vi "Write Settings To VI Controls.vi"(0 "Control In":refnum<vi>, 5 "Control Values":T1[](array[typedef]), 11 "error in":errorcluster) -> (4 "Control Out":refnum<vi>, 15 "error out":errorcluster)   [LabVIEW 2020]
uses:
  <vilib>/addons/analyzer/_analyzerctrls.llb/VIAnCtl Config Control Value.ctl
  <vilib>/Utility/Data Type/NI_Data Type.lvlib
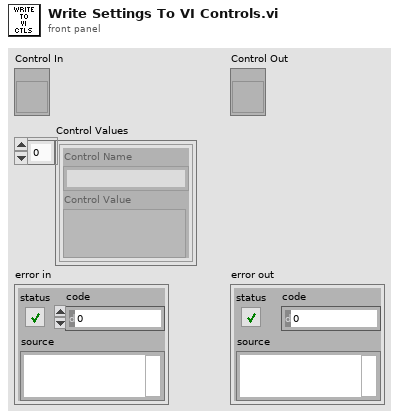
[diagram p1: front panel]
types:
  T1 = typedef "VIAnCtl Config Control Value.ctl" = cluster{"Control Name":string, "Control Value":variant}
  T2 = typedef "NI_Data Type.lvlib/Data Type.ctl" = enum8{"Invalid Type", "Void", "I8", "I16", "I32", "I64", "U8", "U16", "U32", "U64", "Single Float", "Double Float", "Extended Float", "Single Complex", "Double Complex", "Extended Complex", "Enum U8", "Enum U16", "Enum U32", "Enum U64", "Single Float With Unit", "Double Float With Unit", "Extended Float With Unit", "Single Complex with Unit", "Double Complex with Unit", "Extended Complex with Unit", "Boolean", "String", "Path", "Picture", "Tag", "Array", "Cluster", "Variant", "LV Variant", "Waveform", "Timestamp", "Digital Waveform", "Digital Data", "ExpressData", "Refnum", "External Data", "VI", "Poly VI", "LabVIEW Class Instance", "Fixed Point", "Set Collection", "Map Collection"}
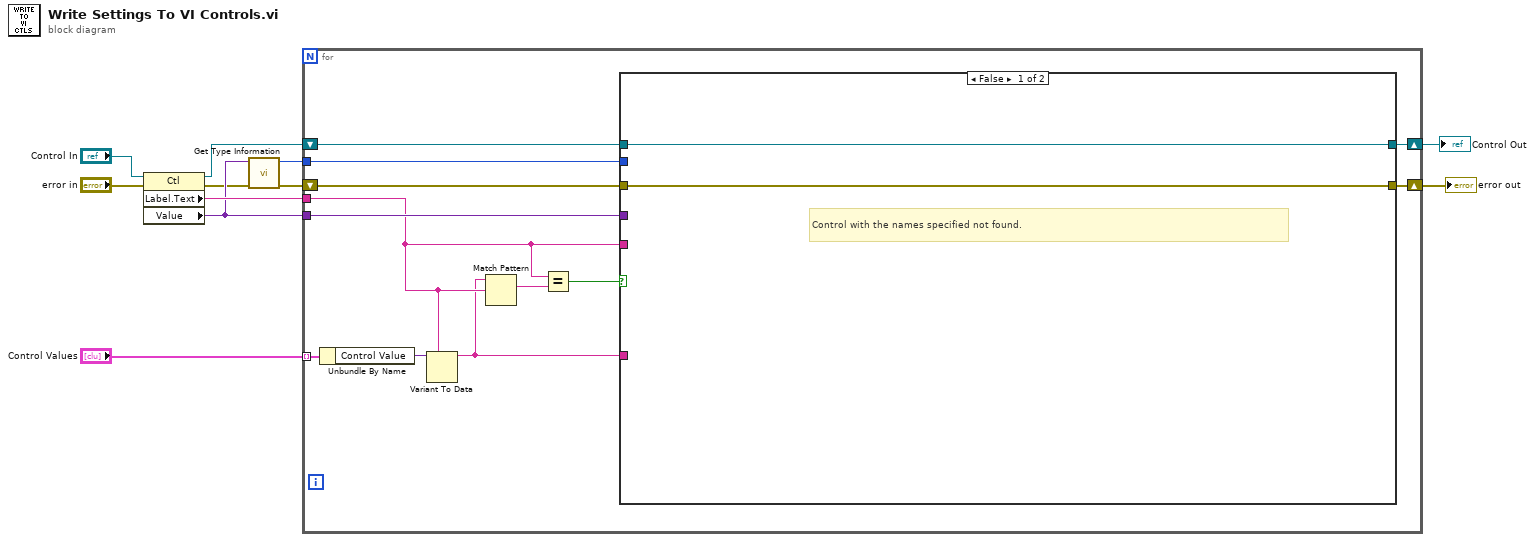
[diagram p0: block diagram]
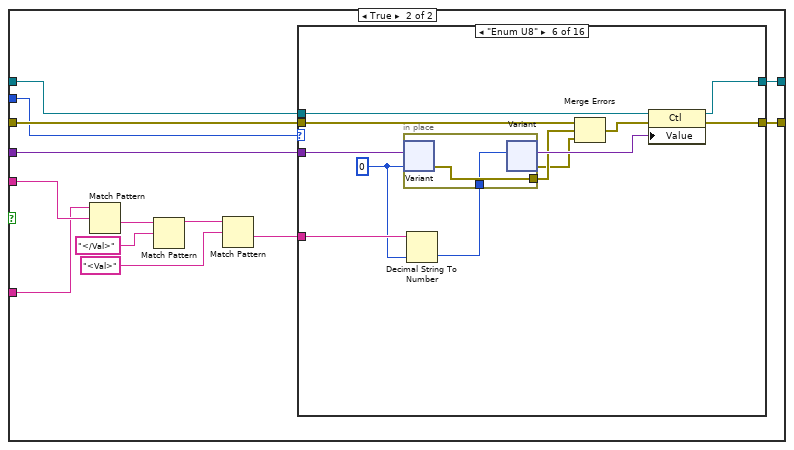
[diagram p2: hidden frame]
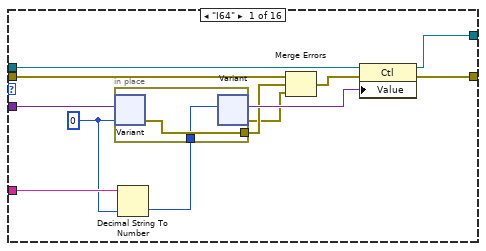
[diagram p3: hidden frame]
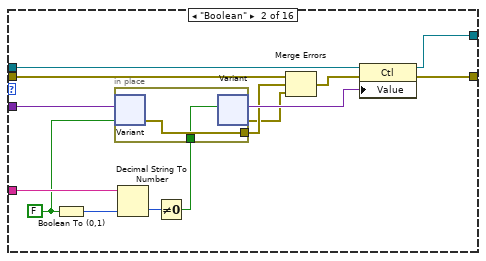
[diagram p4: hidden frame]
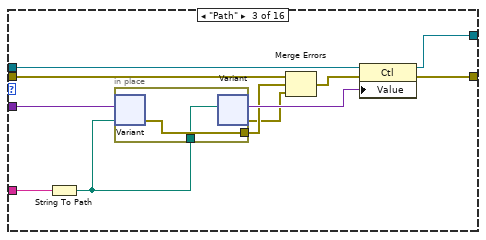
[diagram p5: hidden frame]
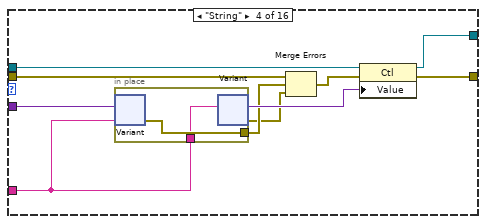
[diagram p6: hidden frame]
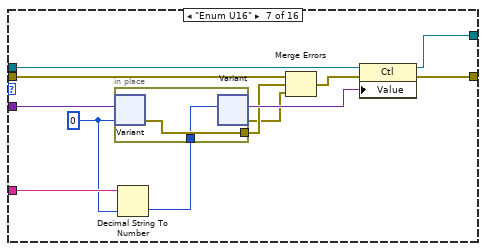
[diagram p8: hidden frame]
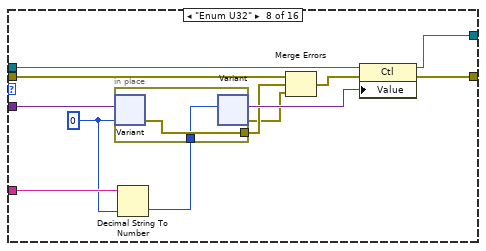
[diagram p9: hidden frame]
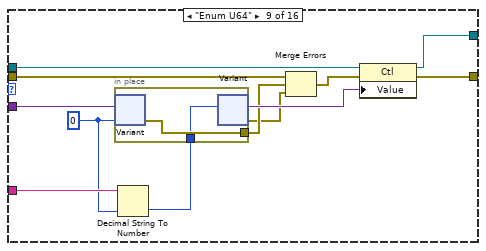
[diagram p10: hidden frame]
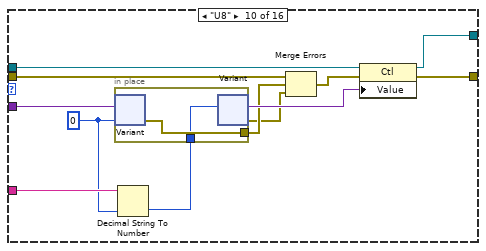
[diagram p11: hidden frame]
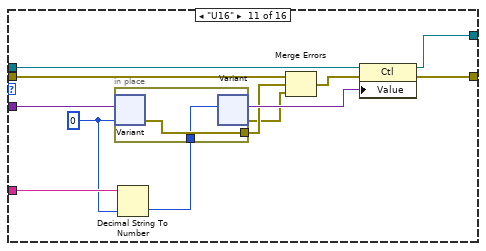
[diagram p12: hidden frame]
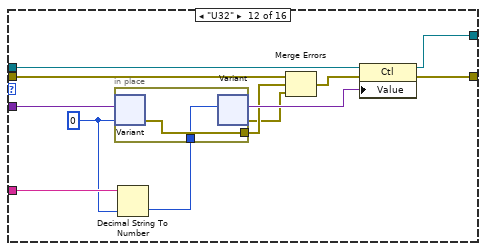
[diagram p13: hidden frame]
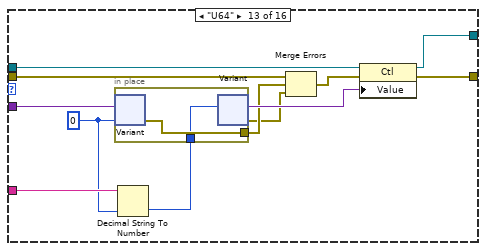
[diagram p14: hidden frame]
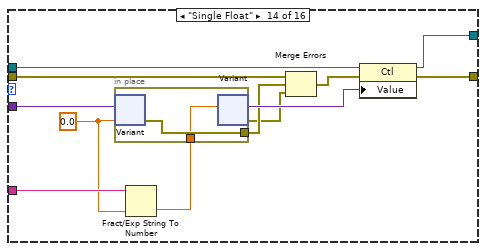
[diagram p15: hidden frame]
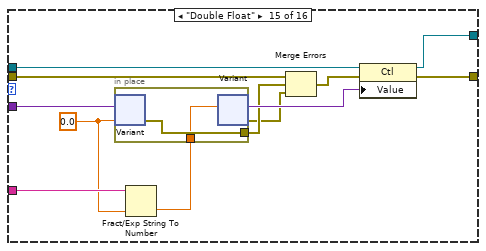
[diagram p16: hidden frame]
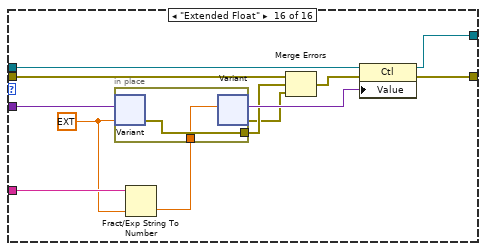
[diagram p17: hidden frame]
diagram:
  n1 = property class="Ctl"(reference="Control In", error in="error in") -> (reference out=w9:refnum<vi>, error out=w5:errorcluster, "Label.Text"=w10:string, "Value"=w6:variant)
  n2 = call <vilib>:"Get Type Information.vi"("error in (no error)"=w5, "variant"=w6) -> ("error out"=w7:errorcluster, "type"=w8:T2)  [unwired: 5 in, 3 out]
  n3 = for {
    shift-right: [w23] -> w2
    shift-left: w7 -> [w19]
    tunnel: "Control Values" -> [w17] mode=indexing
    tunnel: w6 -> [w22]
    tunnel: w8 -> [w21]
    tunnel: w10 -> [w13]
    shift-right: [w15] -> w1
    shift-left: w9 -> [w20]
    n4 = Unbundle By Name(w17) -> ("Control Value"=w14:variant)
    n5 = Variant To Data(type=w13, Variant=w14) -> (data=w12:string)  [unwired: 1 in, 1 out]
    n6 = Match Pattern(string=w12, regular expression=w13) -> (match substring=w16:string)  [unwired: 1 in, 3 out]
    n7 = Equal?(x=w13, y=w16) -> (x = y?=w18:bool)
    n8 = case shown="False" w18 {
      tunnel: [w25 w38] -> w23
      tunnel: w22 -> [_ w37]
      tunnel: w21 -> [_ w27]
      tunnel: w20 -> [w24 w36]
      tunnel: w19 -> [w25 w35]
      tunnel: w12 -> [_ w31]
      tunnel: w13 -> [_ w32]
      tunnel: [w24 w26] -> w15
      frame False {
        # "Control with the names specified not found."
      }
      frame True {
        n9 = Match Pattern(string=w31, regular expression=w32) -> (after substring=w34:string)  [unwired: 1 in, 3 out]
        n10 = Match Pattern(string=w34, regular expression="</Val>") -> (before substring=w30:string)  [unwired: 1 in, 3 out]
        n11 = Match Pattern(string=w30, regular expression="<Val>") -> (after substring=w28:string)  [unwired: 1 in, 3 out]
        n12 = case shown="\"Enum U8\"" w27 {
          tunnel: [w50 w66 w79 w91 w95 w107 w121 w135 w149 w163 w177 w191 w205 w219 w233 w247] -> w38
          tunnel: w37 -> [w49 w65 w78 w90 _ w106 w120 w134 w148 w162 w176 w190 w204 w218 w232 w246]
          tunnel: w36 -> [w48 w64 w77 w89 w94 w105 w119 w133 w147 w161 w175 w189 w203 w217 w231 w245]
          tunnel: w35 -> [w47 w63 w76 w88 w95 w104 w118 w132 w146 w160 w174 w188 w202 w216 w230 w244]
          tunnel: w28 -> [w46 w62 w71 w83 _ w103 w117 w131 w145 w159 w173 w187 w201 w211 w225 w239]
          tunnel: [w39 w53 w69 w82 w94 w96 w110 w124 w138 w152 w166 w180 w194 w208 w222 w236] -> w26
          frame "I64" {
            w40 = i64 0
            n13 = Decimal String To Number(string=w46, default (0L)=w40) -> (number=w41:i64)  [unwired: 1 in, 1 out]
            n14 = in-place {
              in-place-border: [w52] -> w43
              in-place-border: w41 -> [w51]
              n15 = in-place-variant #1(w49, w40) -> (w52:errorcluster)  [unwired: 1 out]
              n16 = in-place-variant #1(w51) -> (w45:variant, w42:errorcluster)
            }
            n17 = Merge Errors(w47, w43, w42) -> (w44:errorcluster)
            n18 = property class="Ctl"(reference=w48, error in=w44, "Value"=w45) -> (reference out=w39:refnum<vi>, error out=w50:errorcluster)
          }
          frame "Boolean" {
            w56 = FALSE ("Boolean")
            n19 = Boolean To (0,1)(Boolean=w56) -> (0, 1=w57:i16)
            n20 = Decimal String To Number(string=w62, default (0L)=w57) -> (number=w55:i16)  [unwired: 1 in, 1 out]
            n21 = Not Equal To 0?(x=w55) -> (x != 0?=w54:bool)
            n22 = in-place {
              in-place-border: [w68] -> w59
              in-place-border: w54 -> [w67]
              n23 = in-place-variant #2(w65, w56) -> (w68:errorcluster)  [unwired: 1 out]
              n24 = in-place-variant #2(w67) -> (w61:variant, w58:errorcluster)
            }
            n25 = Merge Errors(w63, w59, w58) -> (w60:errorcluster)
            n26 = property class="Ctl"(reference=w64, error in=w60, "Value"=w61) -> (reference out=w53:refnum<vi>, error out=w66:errorcluster)
          }
          frame "Path" {
            n27 = String To Path(string=w71) -> (path=w70:path)
            n28 = in-place {
              in-place-border: [w81] -> w73
              in-place-border: w70 -> [w80]
              n29 = in-place-variant #3(w78, w70) -> (w81:errorcluster)  [unwired: 1 out]
              n30 = in-place-variant #3(w80) -> (w75:variant, w72:errorcluster)
            }
            n31 = Merge Errors(w76, w73, w72) -> (w74:errorcluster)
            n32 = property class="Ctl"(reference=w77, error in=w74, "Value"=w75) -> (reference out=w69:refnum<vi>, error out=w79:errorcluster)
          }
          frame "String" {
            n33 = in-place {
              in-place-border: [w93] -> w85
              in-place-border: w83 -> [w92]
              n34 = in-place-variant #4(w90, w83) -> (w93:errorcluster)  [unwired: 1 out]
              n35 = in-place-variant #4(w92) -> (w87:variant, w84:errorcluster)
            }
            n36 = Merge Errors(w88, w85, w84) -> (w86:errorcluster)
            n37 = property class="Ctl"(reference=w89, error in=w86, "Value"=w87) -> (reference out=w82:refnum<vi>, error out=w91:errorcluster)
          }
          frame Default {
            # "Type not handled."
          }
          frame "Enum U8" {
            w97 = u8 0
            n38 = Decimal String To Number(string=w103, default (0L)=w97) -> (number=w98:u8)  [unwired: 1 in, 1 out]
            n39 = in-place {
              in-place-border: [w109] -> w100
              in-place-border: w98 -> [w108]
              n40 = in-place-variant #5(w106, w97) -> (w109:errorcluster)  [unwired: 1 out]
              n41 = in-place-variant #5(w108) -> (w102:variant, w99:errorcluster)
            }
            n42 = Merge Errors(w104, w100, w99) -> (w101:errorcluster)
            n43 = property class="Ctl"(reference=w105, error in=w101, "Value"=w102) -> (reference out=w96:refnum<vi>, error out=w107:errorcluster)
          }
          frame "Enum U16" {
            w111 = u16 0
            n44 = Decimal String To Number(string=w117, default (0L)=w111) -> (number=w112:u16)  [unwired: 1 in, 1 out]
            n45 = in-place {
              in-place-border: [w123] -> w114
              in-place-border: w112 -> [w122]
              n46 = in-place-variant #6(w120, w111) -> (w123:errorcluster)  [unwired: 1 out]
              n47 = in-place-variant #6(w122) -> (w116:variant, w113:errorcluster)
            }
            n48 = Merge Errors(w118, w114, w113) -> (w115:errorcluster)
            n49 = property class="Ctl"(reference=w119, error in=w115, "Value"=w116) -> (reference out=w110:refnum<vi>, error out=w121:errorcluster)
          }
          frame "Enum U32" {
            w125 = u32 0
            n50 = Decimal String To Number(string=w131, default (0L)=w125) -> (number=w126:u32)  [unwired: 1 in, 1 out]
            n51 = in-place {
              in-place-border: [w137] -> w128
              in-place-border: w126 -> [w136]
              n52 = in-place-variant #7(w134, w125) -> (w137:errorcluster)  [unwired: 1 out]
              n53 = in-place-variant #7(w136) -> (w130:variant, w127:errorcluster)
            }
            n54 = Merge Errors(w132, w128, w127) -> (w129:errorcluster)
            n55 = property class="Ctl"(reference=w133, error in=w129, "Value"=w130) -> (reference out=w124:refnum<vi>, error out=w135:errorcluster)
          }
          frame "Enum U64" {
            w139 = u64 0
            n56 = Decimal String To Number(string=w145, default (0L)=w139) -> (number=w140:u64)  [unwired: 1 in, 1 out]
            n57 = in-place {
              in-place-border: [w151] -> w142
              in-place-border: w140 -> [w150]
              n58 = in-place-variant #8(w148, w139) -> (w151:errorcluster)  [unwired: 1 out]
              n59 = in-place-variant #8(w150) -> (w144:variant, w141:errorcluster)
            }
            n60 = Merge Errors(w146, w142, w141) -> (w143:errorcluster)
            n61 = property class="Ctl"(reference=w147, error in=w143, "Value"=w144) -> (reference out=w138:refnum<vi>, error out=w149:errorcluster)
          }
          frame "U8" {
            w153 = u8 0 ("Numeric")
            n62 = Decimal String To Number(string=w159, default (0L)=w153) -> (number=w154:u8)  [unwired: 1 in, 1 out]
            n63 = in-place {
              in-place-border: [w165] -> w156
              in-place-border: w154 -> [w164]
              n64 = in-place-variant #9(w162, w153) -> (w165:errorcluster)  [unwired: 1 out]
              n65 = in-place-variant #9(w164) -> (w158:variant, w155:errorcluster)
            }
            n66 = Merge Errors(w160, w156, w155) -> (w157:errorcluster)
            n67 = property class="Ctl"(reference=w161, error in=w157, "Value"=w158) -> (reference out=w152:refnum<vi>, error out=w163:errorcluster)
          }
          frame "U16" {
            w167 = u16 0 ("Numeric")
            n68 = Decimal String To Number(string=w173, default (0L)=w167) -> (number=w168:u16)  [unwired: 1 in, 1 out]
            n69 = in-place {
              in-place-border: [w179] -> w170
              in-place-border: w168 -> [w178]
              n70 = in-place-variant #10(w176, w167) -> (w179:errorcluster)  [unwired: 1 out]
              n71 = in-place-variant #10(w178) -> (w172:variant, w169:errorcluster)
            }
            n72 = Merge Errors(w174, w170, w169) -> (w171:errorcluster)
            n73 = property class="Ctl"(reference=w175, error in=w171, "Value"=w172) -> (reference out=w166:refnum<vi>, error out=w177:errorcluster)
          }
          frame "U32" {
            w181 = u32 0 ("Numeric")
            n74 = Decimal String To Number(string=w187, default (0L)=w181) -> (number=w182:u32)  [unwired: 1 in, 1 out]
            n75 = in-place {
              in-place-border: [w193] -> w184
              in-place-border: w182 -> [w192]
              n76 = in-place-variant #11(w190, w181) -> (w193:errorcluster)  [unwired: 1 out]
              n77 = in-place-variant #11(w192) -> (w186:variant, w183:errorcluster)
            }
            n78 = Merge Errors(w188, w184, w183) -> (w185:errorcluster)
            n79 = property class="Ctl"(reference=w189, error in=w185, "Value"=w186) -> (reference out=w180:refnum<vi>, error out=w191:errorcluster)
          }
          frame "U64" {
            w195 = u64 0 ("Numeric")
            n80 = Decimal String To Number(string=w201, default (0L)=w195) -> (number=w196:u64)  [unwired: 1 in, 1 out]
            n81 = in-place {
              in-place-border: [w207] -> w198
              in-place-border: w196 -> [w206]
              n82 = in-place-variant #12(w204, w195) -> (w207:errorcluster)  [unwired: 1 out]
              n83 = in-place-variant #12(w206) -> (w200:variant, w197:errorcluster)
            }
            n84 = Merge Errors(w202, w198, w197) -> (w199:errorcluster)
            n85 = property class="Ctl"(reference=w203, error in=w199, "Value"=w200) -> (reference out=w194:refnum<vi>, error out=w205:errorcluster)
          }
          frame "Single Float" {
            w210 = sgl 0.0 ("Numeric")
            n86 = Fract/Exp String To Number(string=w211, default (0 dbl)=w210) -> (number=w209:sgl)  [unwired: 2 in, 1 out]
            n87 = in-place {
              in-place-border: [w221] -> w213
              in-place-border: w209 -> [w220]
              n88 = in-place-variant #13(w218, w210) -> (w221:errorcluster)  [unwired: 1 out]
              n89 = in-place-variant #13(w220) -> (w215:variant, w212:errorcluster)
            }
            n90 = Merge Errors(w216, w213, w212) -> (w214:errorcluster)
            n91 = property class="Ctl"(reference=w217, error in=w214, "Value"=w215) -> (reference out=w208:refnum<vi>, error out=w219:errorcluster)
          }
          frame "Double Float" {
            w224 = 0.0 ("Numeric")
            n92 = Fract/Exp String To Number(string=w225, default (0 dbl)=w224) -> (number=w223:dbl)  [unwired: 2 in, 1 out]
            n93 = in-place {
              in-place-border: [w235] -> w227
              in-place-border: w223 -> [w234]
              n94 = in-place-variant #14(w232, w224) -> (w235:errorcluster)  [unwired: 1 out]
              n95 = in-place-variant #14(w234) -> (w229:variant, w226:errorcluster)
            }
            n96 = Merge Errors(w230, w227, w226) -> (w228:errorcluster)
            n97 = property class="Ctl"(reference=w231, error in=w228, "Value"=w229) -> (reference out=w222:refnum<vi>, error out=w233:errorcluster)
          }
          frame "Extended Float" {
            w238 = ext 0.0 ("Numeric")
            n98 = Fract/Exp String To Number(string=w239, default (0 dbl)=w238) -> (number=w237:ext)  [unwired: 2 in, 1 out]
            n99 = in-place {
              in-place-border: [w249] -> w241
              in-place-border: w237 -> [w248]
              n100 = in-place-variant #15(w246, w238) -> (w249:errorcluster)  [unwired: 1 out]
              n101 = in-place-variant #15(w248) -> (w243:variant, w240:errorcluster)
            }
            n102 = Merge Errors(w244, w241, w240) -> (w242:errorcluster)
            n103 = property class="Ctl"(reference=w245, error in=w242, "Value"=w243) -> (reference out=w236:refnum<vi>, error out=w247:errorcluster)
          }
        }
      }
    }
  }
  "error out" <- w2
  "Control Out" <- w1
